vi "Translate_CartesianVector.vi"(7 "Translation Type":T1, 8 "error in (no error)":errorcluster, 10 "CV 2":refnum<class "CartesianVector.lvclass">, 11 "CV 1":refnum<class "CartesianVector.lvclass">) -> (0 "error out":errorcluster, 3 "CV 1 Translated by CV 2":refnum<class "CartesianVector.lvclass">)   [LabVIEW 2012, in "CartesianVector.lvclass"]
doc: "Translates CV 1 by CV 2 either additively or subtractively depending on the value of Translation Type. The output is the new translated Cartesian Vector."
uses:
  CartesianVector.lvclass
  TypeDefs/TranslationType.ctl
  CartesianVector.lvclass/CartesianVector.ctl
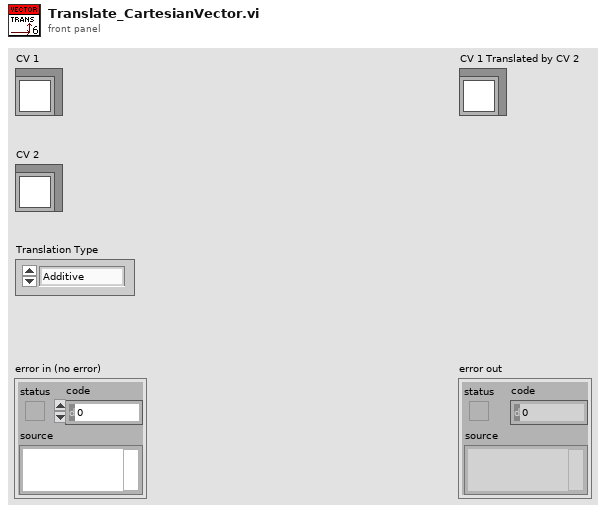
[diagram p1: front panel]
types:
  T1 = typedef "TranslationType.ctl" = enum16{"Additive", "Subtractive"}
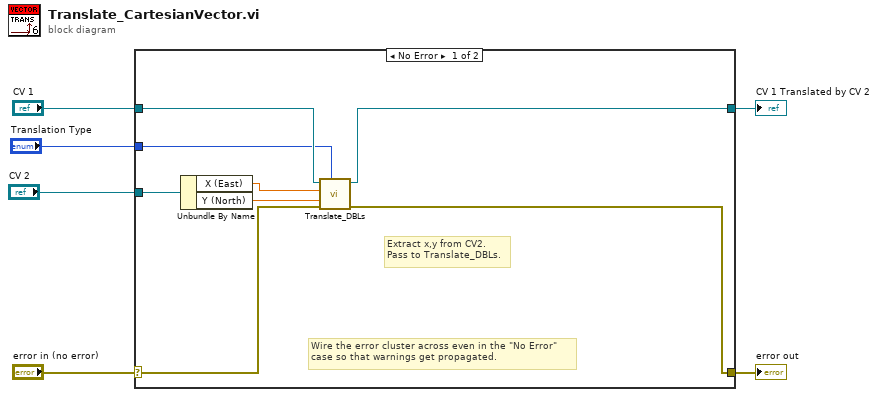
[diagram p0: block diagram]
diagram:
  n1 = case shown="No Error" "error in (no error)" {
    selector: "error in (no error)" -> [w11 w16]
    tunnel: [w10 w16] -> w5
    tunnel: [w8 w15] -> w3
    tunnel: "CV 1" -> [w9 w15]
    tunnel: "CV 2" -> [w14 _]
    tunnel: "Translation Type" -> [w7 _]
    frame No Error {
      # "Extract x,y from CV2.\nPass to Translate_DBLs."
      # "Wire the error cluster across even in the \"No Error\"\ncase so that warnings get propagated."
      n2 = Unbundle By Name(w14) -> ("X (East)"=w13:dbl, "Y (North)"=w12:dbl)
      n3 = call "Translate_DBLs.vi"("Translation Type"=w7, "error in (no error)"=w11, "Y (North)"=w12, "X (East)"=w13, "CartesianVector in"=w9) -> ("error out"=w10:errorcluster, "CartesianVector out"=w8:refnum<class "CartesianVector.lvclass">)  [unwired: 5 in]
    }
    frame Error {
    }
  }
  "error out" <- w5
  "CV 1 Translated by CV 2" <- w3
